vi "log.vi"(4 "Channel":string, 6 "Arguments":map{string, string}(c390), 7 "Time Stamp (now)":timestamp format="%<%x %.3X>T", 8 "error in (no error)":errorcluster, 10 "Message":string, 11 "dataset in":refnum<class "dataset.lvclass">) -> (0 "error out":errorcluster, 3 "dataset out":refnum<class "dataset.lvclass">)   [LabVIEW 2020, in "datasources.lvlib" / "dataset.lvclass"]
uses:
  dataset.lvclass
  dataset.lvclass/dataset.ctl
  Nominal Client.lvclass
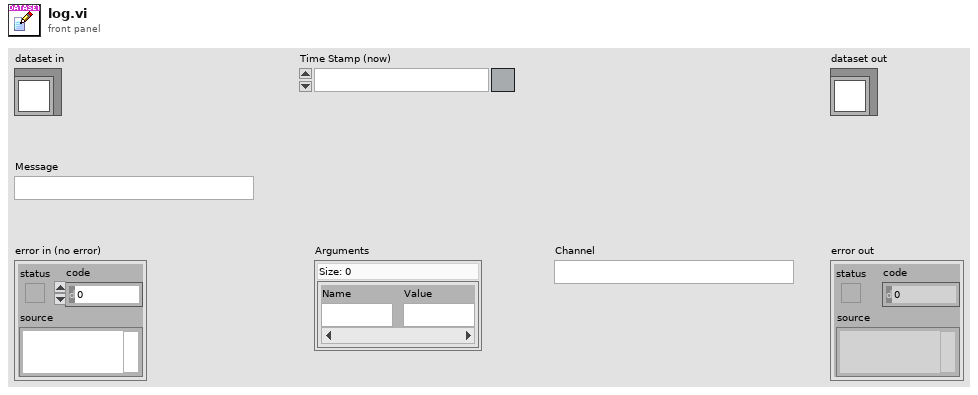
[diagram p1: front panel]
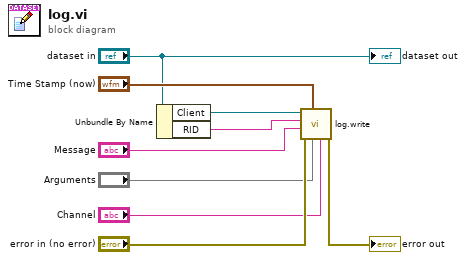
[diagram p0: block diagram]
diagram:
  n1 = Unbundle By Name("dataset in") -> ("Client"=w9:refnum<class "Nominal Client.lvclass">, "RID"=w8:string)
  n2 = call "log.write.vi"("Channel"="Channel", "Arguments"="Arguments", "Time Stamp (now: system time)"="Time Stamp (now)", "error in"="error in (no error)", "Message"="Message", "dataSourceRid"=w8, "Nominal Client in"=w9) -> ("error out"=→"error out":errorcluster)  [unwired: 3 in, 1 out]
  "dataset out" <- "dataset in"
